vi "Create Expanded Terminals.vi"(7 "User App":refnum<vi>, 11 "State":T11={"Worker Library Path"=path "", "Block Label"="", "Types"=[], "Selections"=[], "Icon"={"image type"=0, "image depth"=0, "image"=[], "mask"=[], "colors"=[], "Rectangle"={"left"=0, "top"=0, "right"=0, "bottom"=0}}, "Errors"={"Terminals"=[], "Generate"={"status"=FALSE, "code"=0, "source"=""}, "General"={"status"=FALSE, "code"=0, "source"=""}}, "Calculated Sizes"={"Block Width"=0, "Block Height"=0, "Half Width"=0, "Icon Top"=0, "Icon Bottom"=0, "Label Width"=0, "Half Label"=0, "Label Top"=0, "Text Width"=0, "Half Text"=0, "Text Height"=0, "Label Height"=0, "Expanded Width"=0, "Label Bottom"=0, "Expanded Top"=0, "Expanded Bottom"=0, "Expanded Height"=0, "Min Height"=0, "Max Height"=0}, "Special Terminal Indices"={"Action"=-1, "Init"=-1, "Tag"=-1, "State in"=-1, "State out"=-1, "Error"=-1}, "Terminals"=[]}) -> (3 "Terms":T4[](array[typedef]))   [LabVIEW 2022 SP3, in "FlexBlocks Support.lvlib"]
uses:
  FlexBlocks Support.lvlib
  Flex Block/State.ctl
  Type Descriptor.ctl
  Terminal Direction.ctl
  Value Mode.ctl
  Special Terminal.ctl
  <vilib>/picture/picture.llb/imagedata.ctl
  XNode Errors.ctl
  Calculated Sizes.ctl
  Special Terminal Indices.ctl
  Terminal Status.ctl
  Terminal State.ctl
  Terminal Draw Style.ctl
  <vilib>/XNodeSupport/XNodeTerm4.ctl
  <vilib>/XNodeSupport/XNodeString.ctl
  <vilib>/XNodeSupport/XNodeVariant.ctl
  <vilib>/XNodeSupport/XNodeRect32.ctl
  <vilib>/XNodeSupport/XNodeInt.ctl
  <vilib>/XNodeSupport/XNodeBool.ctl
  <vilib>/XNodeSupport/XNodeTermDirection.ctl
  <vilib>/Utility/Data Type/Type Definitions/Data Type.ctl
  <vilib>/Utility/Data Type/Type Definitions/Type Definition Info.ctl
  <vilib>/XNodeSupport/NI_XNodeSupport.lvlib
  <vilib>/Utility/Data Type/NI_Data Type.lvlib
  Flex Block/Flex Block.xnode
panel:
  out "Array":T3(array[cluster])
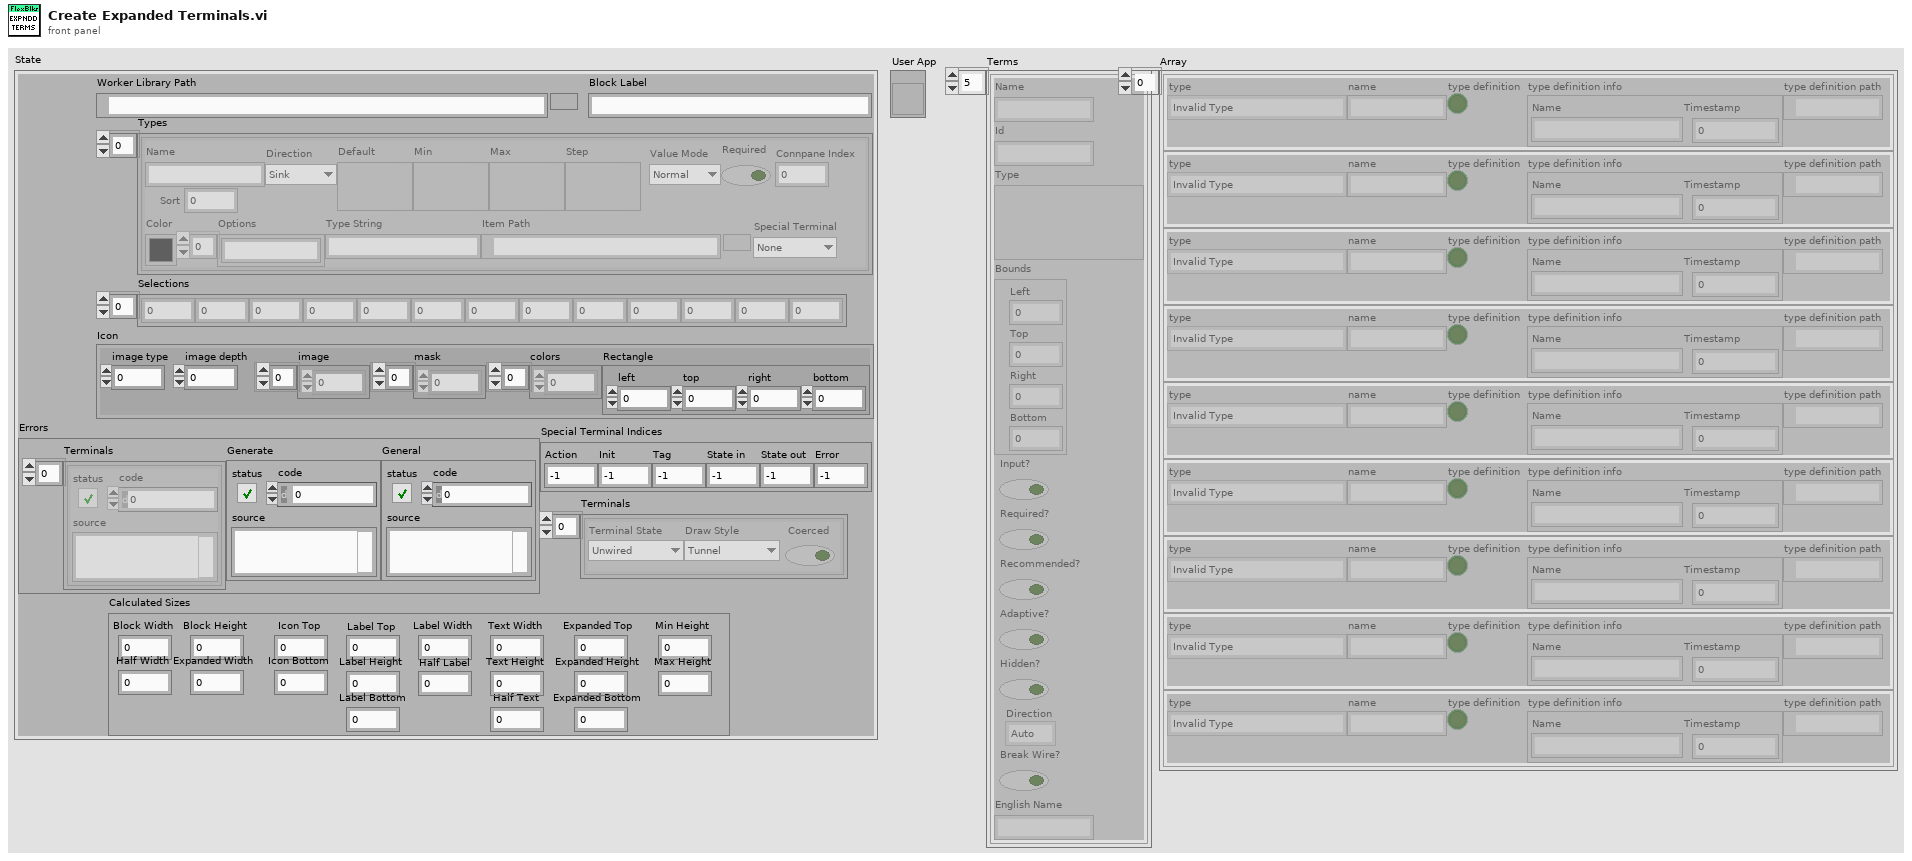
[diagram p1: front panel]
types:
  T1 = typedef "NI_Data Type.lvlib/Data Type.ctl" = enum8{"Invalid Type", "Void", "I8", "I16", "I32", "I64", "U8", "U16", "U32", "U64", "Single Float", "Double Float", "Extended Float", "Single Complex", "Double Complex", "Extended Complex", "Enum U8", "Enum U16", "Enum U32", "Enum U64", "Single Float With Unit", "Double Float With Unit", "Extended Float With Unit", "Single Complex with Unit", "Double Complex with Unit", "Extended Complex with Unit", "Boolean", "String", "Path", "Picture", "Tag", "Array", "Cluster", "Variant", "LV Variant", "Waveform", "Timestamp", "Digital Waveform", "Digital Data", "ExpressData", "Refnum", "External Data", "VI", "Poly VI", "LabVIEW Class Instance", "Fixed Point", "Set Collection", "Map Collection"}
  T2 = typedef "NI_Data Type.lvlib/Type Definition Info.ctl" = cluster{"Name":string, "Timestamp":u32}
  T3 = cluster{"type":T1, "name":string, "type definition":bool, "type definition info":T2, "type definition path":path}[]
  T4 = typedef "NI_XNodeSupport.lvlib/XNodeTerm4.ctl" = cluster{"Name":T5, "Id":T5, "Type":T6, "Bounds":T7, "Input?":T9, "Required?":T9, "Recommended?":T9, "Adaptive?":T9, "Hidden?":T9, "Direction":T10, "Break Wire?":T9, "English Name":T5}
  T5 = typedef "NI_XNodeSupport.lvlib/XNodeString.ctl" = string
  T6 = typedef "NI_XNodeSupport.lvlib/XNodeVariant.ctl" = variant
  T7 = typedef "NI_XNodeSupport.lvlib/XNodeRect32.ctl" = cluster{"Left":T8, "Top":T8, "Right":T8, "Bottom":T8}
  T8 = typedef "NI_XNodeSupport.lvlib/XNodeInt.ctl" = i32
  T9 = typedef "NI_XNodeSupport.lvlib/XNodeBool.ctl" = bool
  T10 = typedef "NI_XNodeSupport.lvlib/XNodeTermDirection.ctl" = enum32{"Auto", "Up", "Down", "Left", "Right", "Center"}
  T11 = typedef "Flex Block.xnode/State.ctl" = cluster{"Worker Library Path":path, "Block Label":string, "Types":T12[], "Selections":i32[], "Icon":T16, "Errors":T17, "Calculated Sizes":T18, "Special Terminal Indices":T19, "Terminals":T20[]}
  T12 = typedef "FlexBlocks Support.lvlib/Type Descriptor.ctl" = cluster{"Name":string, "Direction":T13, "Default":variant, "Min":variant, "Max":variant, "Step":variant, "Value Mode":T14, "Color":u32, "Options":string[], "Type String":string, "Item Path":path, "Required":bool, "Connpane Index":i32, "Special Terminal":T15, "Sort":i32}
  T13 = typedef "FlexBlocks Support.lvlib/Terminal Direction.ctl" = enum16{"Sink", "Source"}
  T14 = typedef "FlexBlocks Support.lvlib/Value Mode.ctl" = enum16{"Normal", "Range", "Select"}
  T15 = typedef "FlexBlocks Support.lvlib/Special Terminal.ctl" = enum16{"None", "Action", "Init", "Tag", "State in", "State out", "Error"}
  T16 = typedef "imagedata.ctl" = cluster{"image type":i32, "image depth":i32, "image":u8[], "mask":u8[], "colors":u32[], "Rectangle":cluster{"left":i16, "top":i16, "right":i16, "bottom":i16}}
  T17 = typedef "FlexBlocks Support.lvlib/XNode Errors.ctl" = cluster{"Terminals":errorcluster[], "Generate":errorcluster, "General":errorcluster}
  T18 = typedef "FlexBlocks Support.lvlib/Calculated Sizes.ctl" = cluster{"Block Width":i32, "Block Height":i32, "Half Width":i32, "Icon Top":i32, "Icon Bottom":i32, "Label Width":i32, "Half Label":i32, "Label Top":i32, "Text Width":i32, "Half Text":i32, "Text Height":i32, "Label Height":i32, "Expanded Width":i32, "Label Bottom":i32, "Expanded Top":i32, "Expanded Bottom":i32, "Expanded Height":i32, "Min Height":i32, "Max Height":i32}
  T19 = typedef "FlexBlocks Support.lvlib/Special Terminal Indices.ctl" = cluster{"Action":i32, "Init":i32, "Tag":i32, "State in":i32, "State out":i32, "Error":i32}
  T20 = typedef "FlexBlocks Support.lvlib/Terminal Status.ctl" = cluster{"Terminal State":T21, "Draw Style":T22, "Coerced":bool}
  T21 = typedef "FlexBlocks Support.lvlib/Terminal State.ctl" = enum16{"Unwired", "BadType", "BadRef", "Channel", "Value", "Control Ref"}
  T22 = typedef "FlexBlocks Support.lvlib/Terminal Draw Style.ctl" = enum16{"Tunnel", "BadType", "BadRef", "Channel", "Value", "Control Ref"}
  T23 = typedef "FlexBlocks Support.lvlib/Size Constants.ctl" = cluster{"Icon Size":i32, "Name H Pad":i32, "Name V Pad":i32, "Max Label Width":i32, "Value Width":i32, "Frame Padding":i32, "Vertical Margin":i32, "Min Width":i32, "Min Height":i32, "Collapsed Spacing":i32, "Terminal Center Offset":i32}
  T24 = cluster{"type":T1, "name":string, "type definition":bool, "type definition info":T2, "type definition path":path}
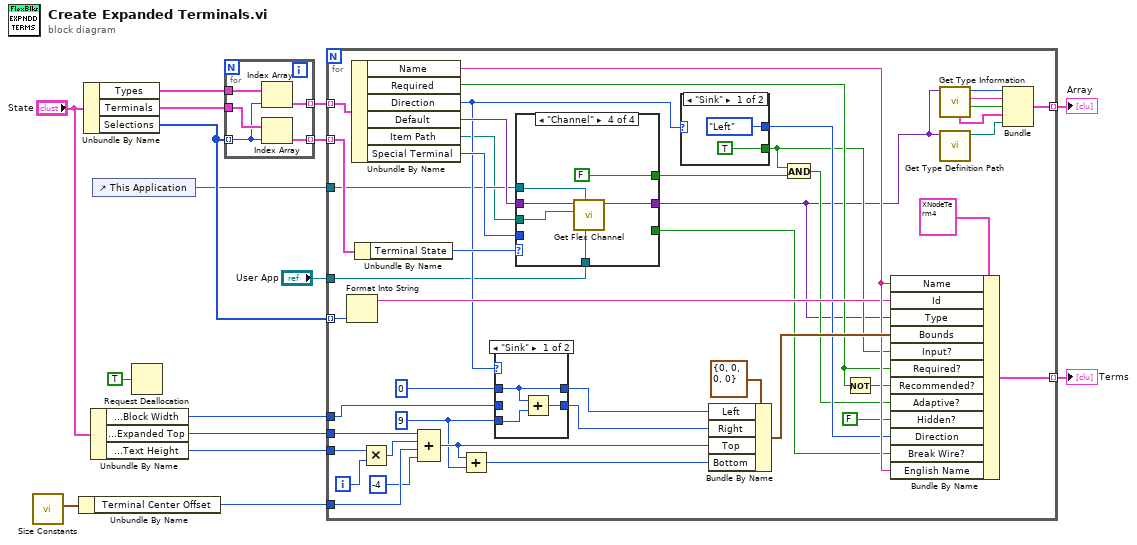
[diagram p0: block diagram]
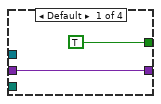
[diagram p2: hidden frame]
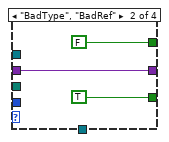
[diagram p3: hidden frame]
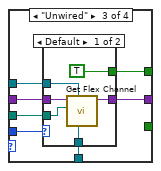
[diagram p4: hidden frame]
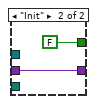
[diagram p5: hidden frame]
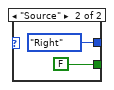
[diagram p6: hidden frame]
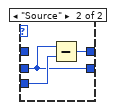
[diagram p7: hidden frame]
diagram:
  n1 = call "Size Constants.vi"() -> ("Size Constants"=w13:T23)  [unwired: 11 in]
  n2 = Unbundle By Name(w13) -> ("Terminal Center Offset"=w9:i32)
  n3 = Unbundle By Name("State") -> ("Types"=w16:T12[], "Terminals"=w6:T20[], "Selections"=w5:i32[])
  n4 = Unbundle By Name("State") -> ("Calculated Sizes.Block Width"=w7:i32, "Calculated Sizes.Expanded Top"=w11:i32, "Calculated Sizes.Text Height"=w10:i32)
  n5 = control-ref of="This Application"() -> (w2:refnum<vi>)
  n6 = Request Deallocation(TRUE ("flag")) -> ()
  n7 = for {
    tunnel: w16 -> [w21]
    tunnel: w5 -> [w18] mode=indexing
    tunnel: [w20] -> w8 mode=indexing
    tunnel: w6 -> [w19]
    tunnel: [w17] -> w4 mode=indexing
    n8 = Index Array(array=w21, index=w18) -> (element=w20:T12)
    n9 = Index Array(array=w19, index=w18) -> (element=w17:T20)
  }
  n10 = for {
    tunnel: [w64] -> w14 mode=indexing
    tunnel: w11 -> [w57]
    tunnel: w10 -> [w53]
    tunnel: w9 -> [w55]
    tunnel: w8 -> [w62] mode=indexing
    tunnel: w7 -> [w61]
    tunnel: w5 -> [w46] mode=indexing
    tunnel: w4 -> [w44] mode=indexing
    tunnel: w2 -> [w31]
    tunnel: [w23] -> w3 mode=indexing
    tunnel: "User App" -> [w22]
    i -> [w63]
    w51 = i16 9 ("Tunnel Size")
    n11 = Format Into String(w46) -> (resulting string=w45:string)  [unwired: 3 in, 1 out]
    n12 = Unbundle By Name(w62) -> ("Name"=w47:string, "Required"=w39:bool, "Direction"=w32:T13, "Default"=w38:variant, "Item Path"=w30:path, "Special Terminal"=w37:T15)
    n13 = Unbundle By Name(w44) -> ("Terminal State"=w41:T21)
    n14 = Multiply(x=w53, y=w63) -> (x*y=w56:i32)
    n15 = Compound Arithmetic op=ADD(w57, w56, w55, -4 ("value")) -> (w52:i32)
    n16 = Add(x=w52, y=w51) -> (x+y=w50:i32)
    n17 = case shown="\"Sink\"" w32 {
      tunnel: 0 ("Calculated Sizes.Block Width") -> [w97 _]
      tunnel: w61 -> [_ w99]
      tunnel: w51 -> [w96 w100]
      tunnel: [w97 w101] -> w49
      tunnel: [w98 w99] -> w48
      frame "Sink" {
        n18 = Add(x=w97, y=w96) -> (x+y=w98:i32)
      }
      frame "Source" {
        n19 = Subtract(x=w99, y=w100) -> (x-y=w101:i32)
      }
    }
    n20 = case shown="\"Channel\"" w41 {
      tunnel: w38 -> [w67 w70 w76 w91]
      tunnel: w37 -> [_ _ w77 _]
      tunnel: [w67 w70 w75 w90] -> w29
      tunnel: [TRUE FALSE w74 FALSE] -> w36
      tunnel: [_ TRUE _ _] -> w33
      tunnel: w31 -> [_ _ w73 w88]
      tunnel: w30 -> [_ _ w72 w87]
      tunnel: w22 -> [_ _ w71 w86]
      frame Default {
      }
      frame "BadType", "BadRef" {
      }
      frame "Unwired" {
        n21 = case shown="Default" w77 {
          tunnel: w76 -> [w83 w85]
          tunnel: [w82 w85] -> w75
          tunnel: [TRUE FALSE] -> w74
          tunnel: w73 -> [w80 _]
          tunnel: w72 -> [w79 _]
          tunnel: w71 -> [w78 _]
          frame Default {
            n22 = call "Get Flex Channel.vi"("User App"=w78, "app"=w80, "Item Path"=w79, "Element Type"=w83) -> ("Channel Type"=w82:variant)  [unwired: 7 in]
          }
          frame "Init" {
          }
        }
      }
      frame "Channel" {
        n23 = call "Get Flex Channel.vi"("User App"=w86, "app"=w88, "Item Path"=w87, "Element Type"=w91) -> ("Channel Type"=w90:variant)  [unwired: 7 in]
      }
    }
    n24 = case shown="\"Sink\"" w32 {
      tunnel: [XNodeTermDirection."Left" ("Direction") XNodeTermDirection."Right" ("Direction")] -> w43
      tunnel: [TRUE FALSE] -> w34
      frame "Sink" {
      }
      frame "Source" {
      }
    }
    n25 = Bundle By Name(cluster=T7 {"Left"=0, "Top"=0, "Right"=0, "Bottom"=0} ("Bounds"), "Left"=w49, "Right"=w48, "Top"=w52, "Bottom"=w50) -> (w58:T7)
    n26 = And(x=w34, y=w36) -> (x .and. y?=w35:bool)
    n27 = Not(x=w39) -> (.not. x?=w40:bool)
    n28 = Bundle By Name(cluster=T4 {"Name"="", "Id"="", "Type"=variant, "Bounds"={"Left"=0, "Top"=0, "Right"=0, "Bottom"=0}, "Input?"=FALSE, "Required?"=FALSE, "Recommended?"=FALSE, "Adaptive?"=FALSE, "Hidden?"=FALSE, "Direction"=enum."Auto", "Break Wire?"=FALSE, "English Name"=""} ("Term 4"), "Name"=w47, "Id"=w45, "Type"=w29, "Bounds"=w58, "Input?"=w34, "Required?"=w39, "Recommended?"=w40, "Adaptive?"=w35, "Hidden?"=T9 FALSE, "Direction"=w43, "Break Wire?"=w33, "English Name"=w47) -> (w64:T4)
    n29 = call <vilib>:"Get Type Information.vi"("variant"=w29) -> ("type definition"=w26:bool, "name"=w27:string, "type"=w28:T1, "type definition info"=w25:T2)  [unwired: 6 in, 1 out]
    n30 = call <vilib>:"Get Type Definition Path.vi"("variant"=w29) -> ("type definition path"=w24:path)  [unwired: 9 in, 1 out]
    n31 = Bundle("type"=w28, "name"=w27, "type definition"=w26, "type definition info"=w25, "type definition path"=w24) -> (w23:T24)  [unwired: 1 in]
  }
  "Terms" <- w14
  "Array" <- w3
